vi "Initialize.vi"(8 "error in (no error)":errorcluster, 11 "Pict Refnum":refnum<vi>) -> (0 "error out":errorcluster, 3 "QMenu Class out":refnum<class "QMenu Class.lvclass">)   [LabVIEW 2020, in "QTab.lvlib" / "QMenu Class.lvclass"]
uses:
  QMenu Class.lvclass
  QMenu Class.lvclass/QMenu Class.ctl
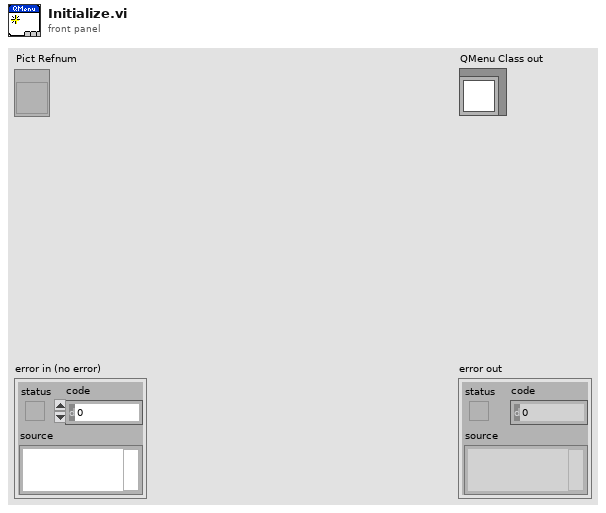
[diagram p1: front panel]
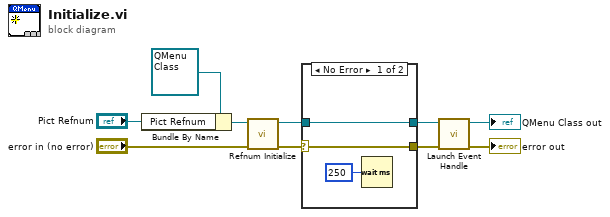
[diagram p0: block diagram]
diagram:
  n1 = Bundle By Name(cluster=refnum<class "QMenu Class.lvclass"> refnum ("QMenu Class out"), "Pict Refnum"="Pict Refnum") -> (w7:refnum<class "QMenu Class.lvclass">)
  n2 = call "Refnum Initialize.vi"("error in (no error)"="error in (no error)", "QMenu Class in"=w7) -> ("error out"=w4:errorcluster, "QMenu Class out"=w2:refnum<class "QMenu Class.lvclass">)  [unwired: 8 in]
  n3 = case shown="No Error" w4 {
    selector: w4 -> [w13 w15]
    tunnel: [w13 w15] -> w3
    tunnel: w2 -> [w12 w14]
    tunnel: [w12 w14] -> w1
    frame No Error {
      n4 = Wait (ms)(milliseconds to wait=u32 250) -> ()  [unwired: 1 out]
    }
    frame Error {
    }
  }
  n5 = call "Launch Event Handle.vi"("error in (no error)"=w3, "QMenu Class in"=w1) -> ("error out"=→"error out":errorcluster, "QMenu Class out"=→"QMenu Class out":refnum<class "QMenu Class.lvclass">)  [unwired: 8 in]
